vi "Create HashingAlgorithm.vi"(8 "error in (no error)":errorcluster, 11 "HashingAlgorithm":T1) -> (0 "error out":errorcluster, 3 "Hashing Algorithm":refnum<k24>)   [LabVIEW 2021, in "dotNET Crypto Utility.lvlib"]
doc: "Create an instance of a .NET hashing algorithm object."
uses:
  dotNET Crypto Utility.lvlib
  HashingAlgorithm.ctl
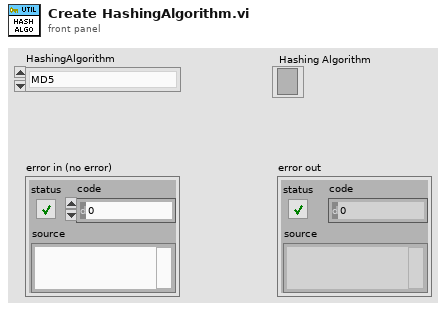
[diagram p1: front panel]
types:
  T1 = typedef "dotNET Crypto Utility.lvlib/HashingAlgorithm.ctl" = enum16{"MD5", "SHA1", "SHA256", "SHA384", "SHA512"}
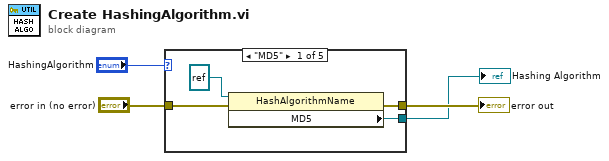
[diagram p0: block diagram]
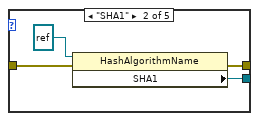
[diagram p2: hidden frame]
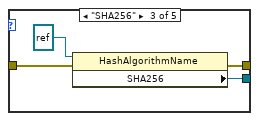
[diagram p3: hidden frame]
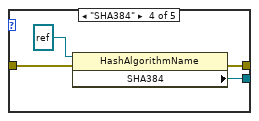
[diagram p4: hidden frame]
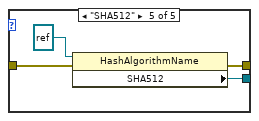
[diagram p5: hidden frame]
diagram:
  n1 = case shown="\"MD5\"" "HashingAlgorithm" {
    tunnel: "error in (no error)" -> [w8 w12 w16 w20 w24]
    tunnel: [w7 w11 w15 w19 w23] -> w3
    tunnel: [w5 w9 w13 w17 w21] -> w1
    frame "MD5" {
      n2 = property class="HashAlgorithmName"(reference=refnum<k24> refnum ("hashAlgorithm"), error in=w8) -> (error out=w7:errorcluster, "MD5"=w5:refnum<k24>)  [unwired: 1 out]
    }
    frame "SHA1" {
      n3 = property class="HashAlgorithmName"(reference=refnum<k24> refnum ("hashAlgorithm"), error in=w12) -> (error out=w11:errorcluster, "SHA1"=w9:refnum<k24>)  [unwired: 1 out]
    }
    frame "SHA256" {
      n4 = property class="HashAlgorithmName"(reference=refnum<k24> refnum ("hashAlgorithm"), error in=w16) -> (error out=w15:errorcluster, "SHA256"=w13:refnum<k24>)  [unwired: 1 out]
    }
    frame "SHA384" {
      n5 = property class="HashAlgorithmName"(reference=refnum<k24> refnum ("hashAlgorithm"), error in=w20) -> (error out=w19:errorcluster, "SHA384"=w17:refnum<k24>)  [unwired: 1 out]
    }
    frame "SHA512" {
      n6 = property class="HashAlgorithmName"(reference=refnum<k24> refnum ("hashAlgorithm"), error in=w24) -> (error out=w23:errorcluster, "SHA512"=w21:refnum<k24>)  [unwired: 1 out]
    }
  }
  "error out" <- w3
  "Hashing Algorithm" <- w1
